vi "Set IPS120 Control.vi"(8 "Error In":errorcluster, 10 "Command string":string, 11 "VISA resource name":refnum<visa-resource-name>) -> (0 "Error Out":errorcluster, 3 "VISA resource name out":refnum<visa-resource-name>)   [LabVIEW 2018]
panel:
  out "read buffer 3":string
  out "read buffer 2":string
  out "substring":string
  out "read buffer":string
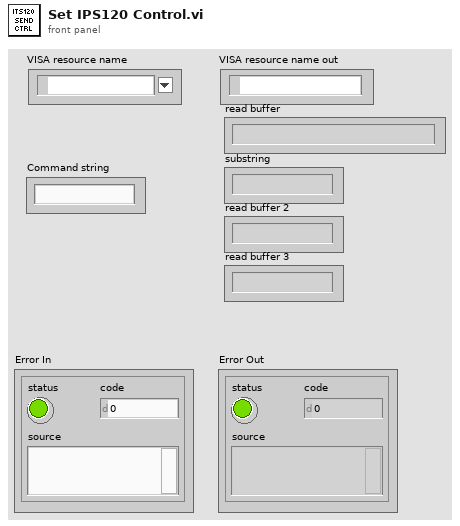
[diagram p1: front panel]
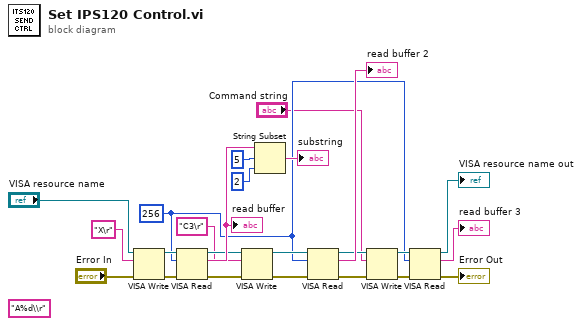
[diagram p0: block diagram]
diagram:
  w3 = u32 256 ("byte count")
  (unwired) "A%d\\r" ("format string")
  n1 = VISA Write(VISA resource name="VISA resource name", write buffer="X\r", error in (no error)="Error In") -> (VISA resource name out=w21:refnum<visa-resource-name>, error out=w23:errorcluster)  [unwired: 1 out]
  n2 = VISA Read(VISA resource name=w21, byte count=w3, error in (no error)=w23) -> (VISA resource name out=w14:refnum<visa-resource-name>, read buffer=w19:string, error out=w15:errorcluster)  [unwired: 1 out]
  "read buffer" <- w19
  n3 = VISA Write(VISA resource name=w14, write buffer="C3\r", error in (no error)=w15) -> (VISA resource name out=w12:refnum<visa-resource-name>, error out=w13:errorcluster)  [unwired: 1 out]
  n4 = String Subset(string=w19, offset (0)=5 ("length (rest)"), length (rest)=2 ("length (rest)")) -> (substring=→"substring":string)
  n5 = VISA Read(VISA resource name=w12, byte count=w3, error in (no error)=w13) -> (VISA resource name out=w7:refnum<visa-resource-name>, read buffer=→"read buffer 2":string, error out=w6:errorcluster)  [unwired: 1 out]
  n6 = VISA Write(VISA resource name=w7, write buffer="Command string", error in (no error)=w6) -> (VISA resource name out=w9:refnum<visa-resource-name>, error out=w8:errorcluster)  [unwired: 1 out]
  n7 = VISA Read(VISA resource name=w9, byte count=w3, error in (no error)=w8) -> (VISA resource name out=→"VISA resource name out":refnum<visa-resource-name>, read buffer=→"read buffer 3":string, error out=→"Error Out":errorcluster)  [unwired: 1 out]
